vi "Build Data URI.vi"(8 "error in (no error)":errorcluster, 11 "OpenHW in":refnum<class "OpenHW.lvclass">) -> (0 "error out":errorcluster, 3 "OpenHW out":refnum<class "OpenHW.lvclass">)   [LabVIEW 2022 SP3, in "open-hw-mon-lv.lvlib" / "OpenHW.lvclass"]
uses:
  OpenHW.lvclass
  OpenHW.lvclass/OpenHW.ctl
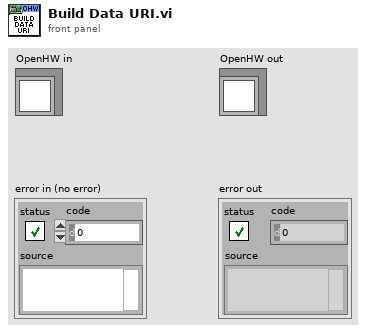
[diagram p1: front panel]
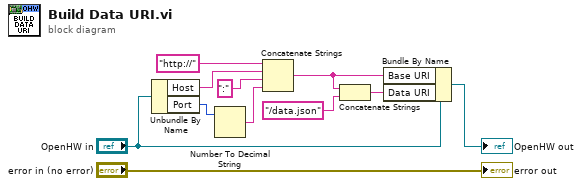
[diagram p0: block diagram]
diagram:
  n1 = Unbundle By Name("OpenHW in") -> ("Host"=w7:string, "Port"=w9:u16)
  n2 = Number To Decimal String(number=w9) -> (decimal integer string=w5:string)  [unwired: 1 in]
  n3 = Concatenate Strings("http://" ("string"), w7, ":" ("string"), w5) -> (w3:string)
  n4 = Concatenate Strings(w3, "/data.json" ("string")) -> (w1:string)
  n5 = Bundle By Name(cluster="OpenHW in", "Base URI"=w3, "Data URI"=w1) -> (→"OpenHW out":refnum<class "OpenHW.lvclass">)
  "error out" <- "error in (no error)"
